vi "XMLparser.vi"(1 "parameters":string[](array[string]), 2 "XML File Path":path) -> (0 "toArrayParser":string[][](array[string]))   [LabVIEW 2009]
uses:
  <vilib>/xml/NI_XML.lvlib
  Program Files/National Instruments/LabVIEW 2009/resource/objmgr/DOMUserDefRef.rc
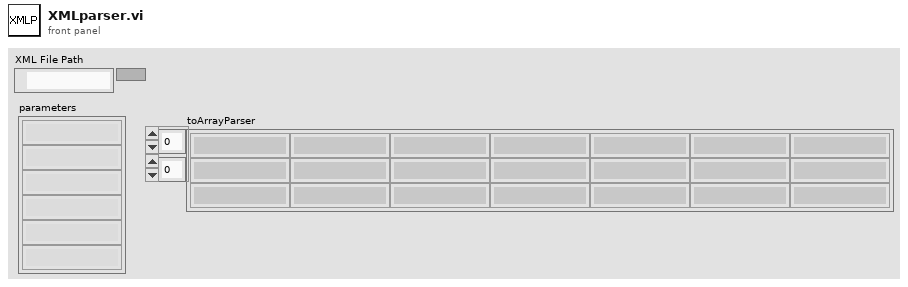
[diagram p1: front panel]
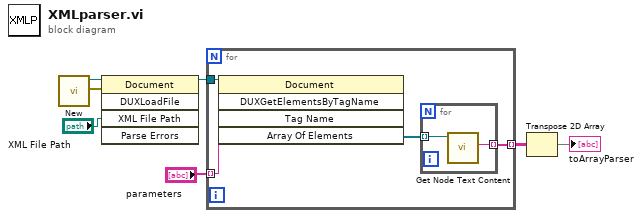
[diagram p0: block diagram]
diagram:
  n1 = call <vilib>:"New.vi"() -> ("error out"=w6:errorcluster, "DOM document out"=w7:refnum<k20>)  [unwired: 8 in]
  n2 = invoke class="Document" method="DUXLoadFile"(reference=w7, error in=w6, "XML File Path"="XML File Path") -> (reference out=w3:refnum<k20>)  [unwired: 2 in, 4 out]
  n3 = for {
    tunnel: "parameters" -> [w11] mode=indexing
    tunnel: [w10] -> w4 mode=indexing
    tunnel: w3 -> [w9]
    n4 = invoke class="Document" method="DUXGetElementsByTagName"(reference=w9, "Tag Name"=w11) -> ("Array Of Elements"=w8:refnum<k20>[])  [unwired: 3 in, 4 out]
    n5 = for {
      tunnel: w8 -> [w13] mode=indexing
      tunnel: [w12] -> w10 mode=indexing
      n6 = call <vilib>:"Get Node Text Content.vi"("node in"=w13) -> ("node text"=w12:string)  [unwired: 8 in, 2 out]
    }
  }
  n7 = Transpose 2D Array(2D array=w4) -> (transposed array=→"toArrayParser":string[][])
